vi "copy area.vi"   [LabVIEW 2012]
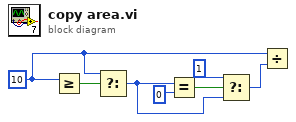
[diagram p0: block diagram]
diagram:
  w2 = u8 10 ("y")
  n1 = Greater Or Equal?(x=w2) -> (x >= y?=w3:bool)  [unwired: 1 in]
  n2 = Select(t=w2, s=w3) -> (s? t:f=w1:u8)  [unwired: 1 in]
  n3 = Equal?(x=w1, y=u8 0) -> (x = y?=w6:bool)
  n4 = Select(t=1, s=w6, f=w1) -> (s? t:f=w4:i32)
  n5 = Divide(x=w2, y=w4) -> ()  [unwired: 1 out]
